vi "ComputeRectROI.vi"(1 "Rectangles":T1(array[cluster]) {"Corners"."Y" format="%.2f"; "Corners"."X" format="%.2f"}) -> (0 "Rectangle":T2 {"Rotation" min=-90.0 max=90.0 step=1.0 format="%.2f"; "Left" scale=0.0..1024.0; "Right" scale=0.0..1024.0})   [LabVIEW 2017]
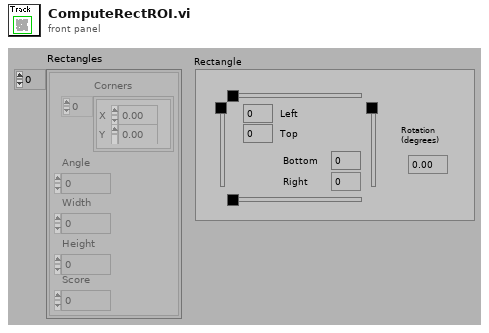
[diagram p1: front panel]
types:
  T1 = cluster{"Corners":cluster{"X":sgl, "Y":sgl}[], "Angle":dbl, "Width":dbl, "Height":dbl, "Score":dbl}[]
  T2 = typedef "IMAQ Rectangle" = cluster{"Left":i32, "Top":i32, "Right":i32, "Bottom":i32, "Rotation":dbl}
  T3 = cluster{"Corners":cluster{"X":sgl, "Y":sgl}[], "Angle":dbl, "Width":dbl, "Height":dbl, "Score":dbl}
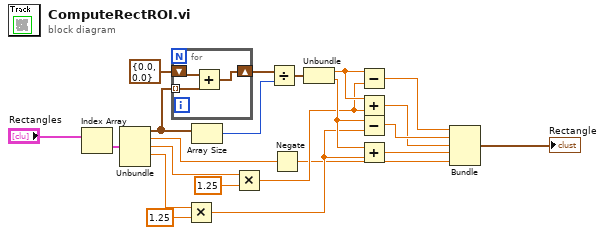
[diagram p0: block diagram]
diagram:
  n1 = Index Array(array="Rectangles") -> (element=w22:T3)  [unwired: 1 in]
  n2 = Unbundle(w22) -> ("Corners"=w16:cluster{"X":sgl, "Y":sgl}[], "Angle"=w14:dbl, "Width"=w12:dbl, "Height"=w11:dbl)  [unwired: 1 out]
  n3 = for {
    tunnel: w16 -> [w25] mode=indexing
    shift-right: [w23] -> w17
    shift-left: cluster{"X":sgl, "Y":sgl} {"X"=0.0, "Y"=0.0} -> [w24]
    n4 = Add(x=w24, y=w25) -> (x+y=w23:cluster{"X":sgl, "Y":sgl})
  }
  n5 = Multiply(x=w11, y=1.25) -> (x*y=w7:dbl)
  n6 = Array Size(array=w16) -> (size(s)=w15:i32)
  n7 = Multiply(x=w12, y=1.25) -> (x*y=w6:dbl)
  n8 = Divide(x=w17, y=w15) -> (x/y=w10:cluster{"X":sgl, "Y":sgl})
  n9 = Negate(x=w14) -> (-x=w1:dbl)
  n10 = Unbundle(w10) -> ("X"=w9:sgl, "Y"=w8:sgl)
  n11 = Subtract(x=w9, y=w6) -> (x-y=w4:dbl)
  n12 = Add(x=w9, y=w6) -> (x+y=w2:dbl)
  n13 = Subtract(x=w8, y=w7) -> (x-y=w3:dbl)
  n14 = Add(x=w8, y=w7) -> (x+y=w5:dbl)
  n15 = Bundle(w4, w3, w2, w5, w1) -> (→"Rectangle":cluster{dbl, dbl, dbl, dbl, dbl})  [unwired: 1 in]
